vi "Error collector.vi"(8 "error list":errorcluster, 11 "error in":errorcluster) -> (2 "error out":errorcluster)   [LabVIEW 2018]
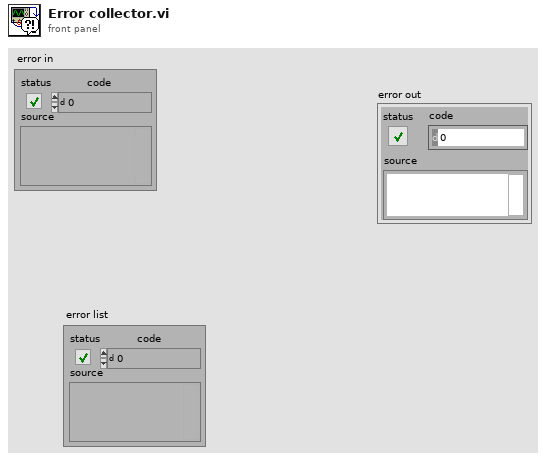
[diagram p1: front panel]
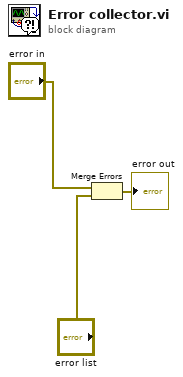
[diagram p0: block diagram]
diagram:
  n1 = Merge Errors("error in", "error list") -> (→"error out":errorcluster)
